vi "绝对偏差百分比出数.vi"(0 "基准值":dbl, 2 "原始值":dbl, 3 "绝对偏差值":dbl) -> (6 "取值输出":dbl, 7 "随机值？":bool)   [LabVIEW 2016, in "random number.lvlib"]
uses:
  random number.lvlib
panel:
  out "已强制转换(x)":dbl
  out "下限":dbl
  out "上限":dbl
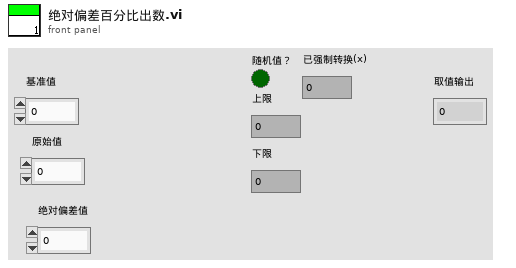
[diagram p1: front panel]
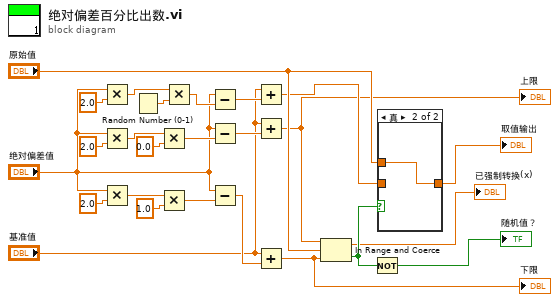
[diagram p0: block diagram]
diagram:
  n1 = Multiply(x="绝对偏差值", y=2.0) -> (x*y=w22:dbl)
  n2 = Multiply(x="绝对偏差值", y=2.0) -> (x*y=w19:dbl)
  n3 = Multiply(x="绝对偏差值", y=2.0) -> (x*y=w14:dbl)
  n4 = Random Number (0-1)() -> (number: 0 to 1=w25:dbl)
  n5 = Multiply(x=w19, y=0.0) -> (x*y=w18:dbl)
  n6 = Multiply(x=w14, y=1.0) -> (x*y=w15:dbl)
  n7 = Multiply(x=w22, y=w25) -> (x*y=w24:dbl)
  n8 = Subtract(x="绝对偏差值", y=w24) -> (x-y=w23:dbl)
  n9 = Subtract(x="绝对偏差值", y=w18) -> (x-y=w11:dbl)
  n10 = Subtract(x="绝对偏差值", y=w15) -> (x-y=w4:dbl)
  n11 = Add(x="基准值", y=w23) -> (x+y=w7:dbl)
  n12 = Add(x="基准值", y=w11) -> (x+y=w2:dbl)
  "上限" <- w2
  n13 = Add(x="基准值", y=w4) -> (x+y=w1:dbl)
  "下限" <- w1
  n14 = In Range and Coerce(upper limit=w2, x="原始值", lower limit=w1) -> (coerced(x)=→"已强制转换(x)":dbl, In Range?=w10:bool)
  n15 = Not(x=w10) -> (.not. x?=→"随机值？":bool)
  n16 = case shown="真" w10 {
    tunnel: "原始值" -> [_ w27]
    tunnel: [w26 w27] -> w8
    tunnel: w7 -> [w26 _]
    frame False {
    }
    frame True {
    }
  }
  "取值输出" <- w8
